vi "DAQ_PW_Calibration.vi"(6 "waveform in":waveform(sgl), 9 "data":waveform(dbl), 10 "MA/UA":bool, 11 "calibration":dbl format="%#_13g") -> (3 "waveform out 2":waveform(sgl))   [LabVIEW 2015]
uses:
  uPower-Kit2/Range_Shunt_selector.ctl
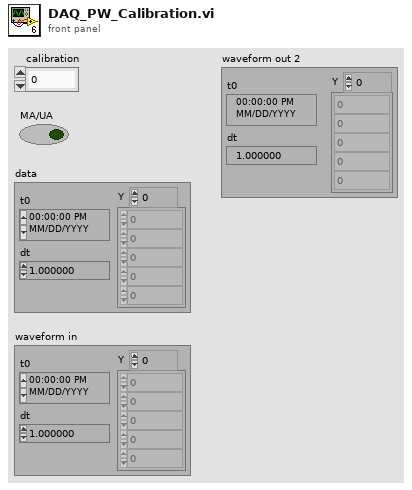
[diagram p1: front panel]
types:
  T1 = typedef "Range_Shunt_selector.ctl" = enum16{"uA Range  Rs = 3.3ohm", "mA Range Rs = 3.3ohm", "mA Range Rs = 1ohm", "mA Range Rs = 1ohm - X2"}
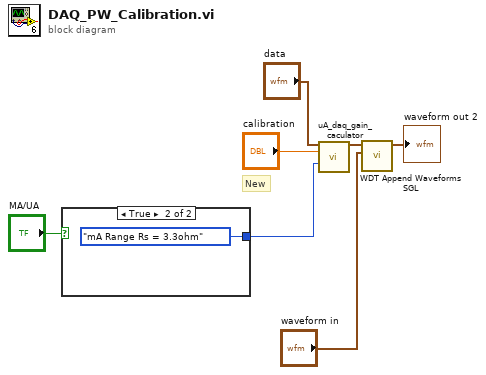
[diagram p0: block diagram]
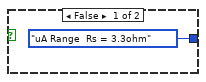
[diagram p2: hidden frame]
diagram:
  # "New"
  n1 = case shown="True" "MA/UA" {
    tunnel: [Range_Shunt_selector."uA Range  Rs = 3.3ohm" ("Range - Shunts") Range_Shunt_selector."mA Range Rs = 3.3ohm" ("Range - Shunts")] -> w4
    frame False {
    }
    frame True {
    }
  }
  n2 = call "uA_daq_gain_caculator.vi"("Waveform Chart in"="data", "Calib_value"="calibration", "Range - Shunts"=w4) -> ("Waveform out"=w1:waveform(dbl))  [unwired: 12 in]
  n3 = call "WDT Append Waveforms SGL.vi"("waveform B"="waveform in", "waveform A"=w1) -> ("waveform out"=→"waveform out 2":waveform(sgl))  [unwired: 8 in, 1 out]
